vi "Handle Suite Results.vi"(8 "error in (no error)":errorcluster, 10 "Test Suite Result":refnum<class "Test Suite Result.lvclass">, 11 "Test Runner In":refnum<class "Test Runner.lvclass">) -> (0 "error out":errorcluster, 3 "Test Runner Out":refnum<class "Test Runner.lvclass">)   [LabVIEW 2020, in "Test Runner.lvclass"]
doc: "Send Suite Results to report generator process."
uses:
  Test Runner.lvclass
  Result Classes/Test Suite Result/Test Suite Result.lvclass
  Test Runner.lvclass/Test Runner.ctl
  Result Collector/Result Collector.lvclass/Result Collector.ctl
  Result Collector/Result Collector.lvclass
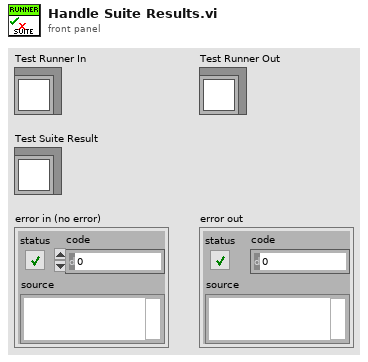
[diagram p1: front panel]
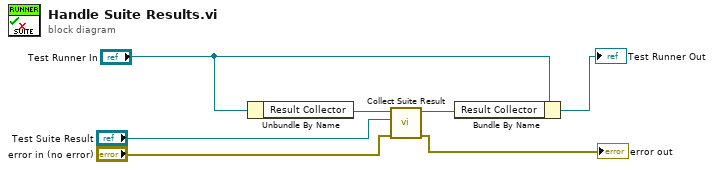
[diagram p0: block diagram]
diagram:
  n1 = Unbundle By Name("Test Runner In") -> ("Result Collector"=w3:refnum<class "Result Collector.lvclass">)
  n2 = call "Collect Suite Result.vi"("error in (no error)"="error in (no error)", "Test Suite Result"="Test Suite Result", "Report Generator In"=w3) -> ("error out"=→"error out":errorcluster, "Report Generator Out"=w4:refnum<class "Result Collector.lvclass">)  [unwired: 7 in]
  n3 = Bundle By Name(cluster="Test Runner In", "Result Collector"=w4) -> (→"Test Runner Out":refnum<class "Test Runner.lvclass">)
